vi "Link Control References.vi"(8 "error in":errorcluster, 10 "Control Map":T1[](array[typedef]), 11 "Multimeter in":refnum<class "Multimeter.lvclass">) -> (0 "error out":errorcluster, 3 "Multimeter out":refnum<class "Multimeter.lvclass">)   [LabVIEW 2019, in "Multimeter.lvlib" / "Multimeter.lvclass"]
uses:
  Library/Multimeter.lvclass
  builds/Instruments/Instruments.lvlibp/Custom Controls/Control Element.ctl
  Library/Multimeter.lvclass/Multimeter.ctl
  builds/Instruments/Instruments.lvlibp/Library/Instruments.lvclass
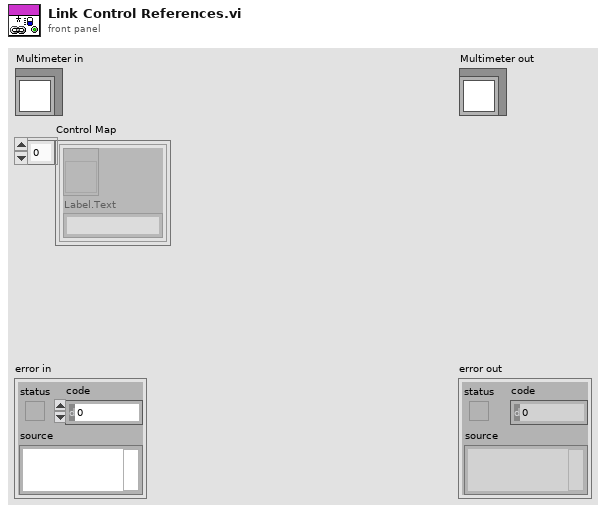
[diagram p1: front panel]
types:
  T1 = typedef "Instruments.lvlibp/Instruments.lvclass/Control Element.ctl" = cluster{refnum<vi>, "Label.Text":string}
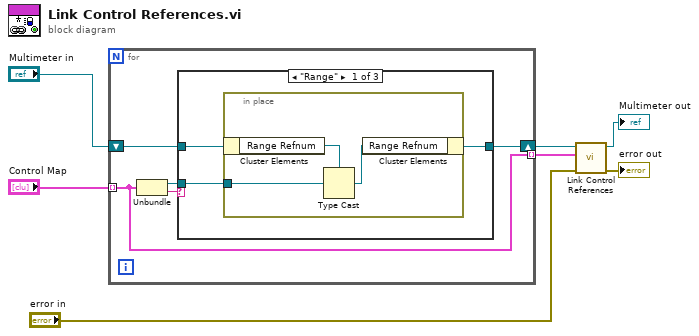
[diagram p0: block diagram]
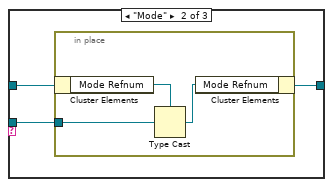
[diagram p2: hidden frame]
diagram:
  n1 = for {
    shift-right: [w9] -> w5
    shift-left: "Multimeter in" -> [w10]
    tunnel: "Control Map" -> [w8] mode=indexing
    tunnel: [w8] -> w3 mode=indexing
    n2 = Unbundle(w8) -> (w11:refnum<vi>, "Label.Text"=w12:string)
    n3 = case shown="\"Range\"" w12 {
      tunnel: w11 -> [w13 w19 _]
      tunnel: w10 -> [w15 w21 w25]
      tunnel: [w14 w20 w25] -> w9
      frame "Range" {
        n4 = in-place {
          in-place-border: w13 -> [w17]
          n5 = in-place-cluster #1(w15) -> ("Range Refnum"=w18:refnum<vi>)
          n6 = Type Cast(type=w18, x=w17) -> (*(type *) &x=w16:refnum<vi>)
          n7 = in-place-cluster #1("Range Refnum"=w16) -> (w14:refnum<class "Multimeter.lvclass">)
        }
      }
      frame "Mode" {
        n8 = in-place {
          in-place-border: w19 -> [w23]
          n9 = in-place-cluster #2(w21) -> ("Mode Refnum"=w24:refnum<vi>)
          n10 = Type Cast(type=w24, x=w23) -> (*(type *) &x=w22:refnum<vi>)
          n11 = in-place-cluster #2("Mode Refnum"=w22) -> (w20:refnum<class "Multimeter.lvclass">)
        }
      }
      frame Default {
      }
    }
  }
  n12 = call-parent "Link Control References.vi"("error in (no error)"="error in", "Control Map"=w3, "Instruments in"=w5) -> ("error out"=→"error out":errorcluster, "Instruments out"=→"Multimeter out":refnum<class "Multimeter.lvclass">)  [unwired: 7 in]
